vi "Bsp_case_structure.vi"() -> ()   [LabVIEW 2013]
panel:
  out "Ergebnis":dbl
  in  "y":dbl
  in  "x":dbl
  in  "subtrahieren":bool
  in  "addieren":bool
  in  "Stopp":bool
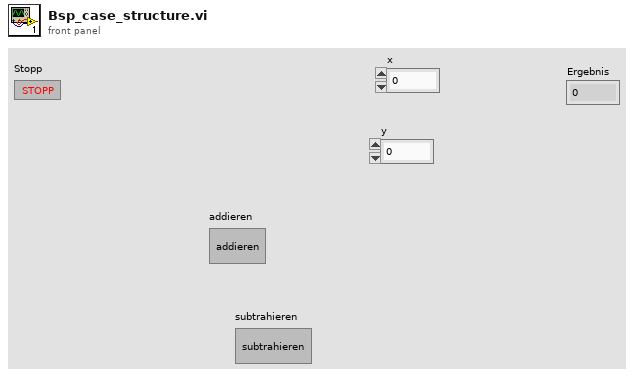
[diagram p1: front panel]
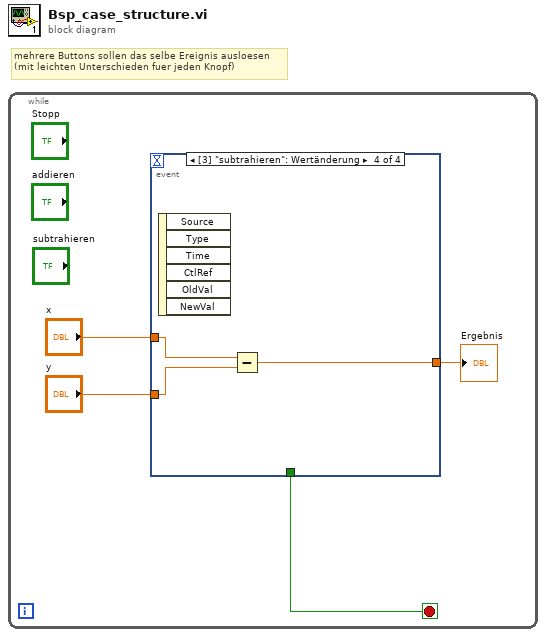
[diagram p0: block diagram]
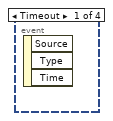
[diagram p2: hidden frame]
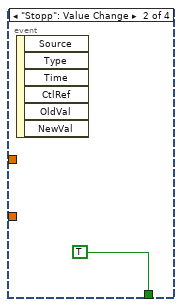
[diagram p3: hidden frame]
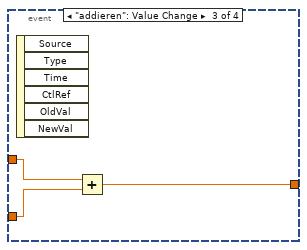
[diagram p4: hidden frame]
diagram:
  # "mehrere Buttons sollen das selbe Ereignis ausloesen\n(mit leichten Unterschieden fuer jeden Knopf)"
  n1 = while {
    stop <- w4 stop-if-true
    n2 = event shown="[3] \"subtrahieren\": Wertänderung" {
      selector: _ -> [_ _ _ _]
      dyn-events: _ -> [_ _ _ _]
      timeout: _ -> [_ _ _ _]
      tunnel: [_ TRUE _ _] -> w4
      tunnel: "y" -> [_ _ w7 w10]
      tunnel: "x" -> [_ _ w8 w11]
      tunnel: [_ _ w6 w9] -> w1
      event Timeout {
        n3 = event-data() -> ()  [unwired: 1 in, 3 out]
      }
      event "Stopp": Value Change {
        n4 = event-data() -> ()  [unwired: 1 in, 6 out]
      }
      event "addieren": Value Change {
        n5 = event-data() -> ()  [unwired: 1 in, 6 out]
        n6 = Add(x=w8, y=w7) -> (x+y=w6:dbl)
      }
      event "subtrahieren": Value Change {
        n7 = event-data() -> ()  [unwired: 1 in, 6 out]
        n8 = Subtract(x=w11, y=w10) -> (x-y=w9:dbl)
      }
    }
    "Ergebnis" <- w1
  }
